vi "E816_Piezo_ctrl_Sereial_mvmnt.vi"() -> ()   [LabVIEW 2016]
doc: "This VI demonstrates how to initialize an E-816 system, how to move an axis and how to query for the position value of this axis.\n\nIn this example the E-816 is connected through COM port 1 with baudrate 57600. The VI runs E816_Configuration_Setup.vi with these specified settings, moves the first axis relative to its current position, waits for the movement to finish and reads the position of the axis and the error status of the controller. The diagram shows how to combine the driver VIs for these tasks. \n\nFor an example of how to command multiple axes through an USB connection see E816_Sample_ Application_1a.vi\n\nWarning: Before running this VI, modify the interface settings on the block diagram to reflect your configuration. The predefined settings provided with the VI probably do not match your system."
panel:
  out "Position":dbl[](array[numeric]) format="%.6f"
  out "First conn. axis":string[](array[string])
  in  "Step values 2":dbl[](array[numeric])=[0.01]
  in  "move":bool
  in  "stop":bool
  in  "error in":errorcluster
  out "Running":bool caption="Configuration_Setup.vi is running"
  out "error out":errorcluster
  out "Identification":string
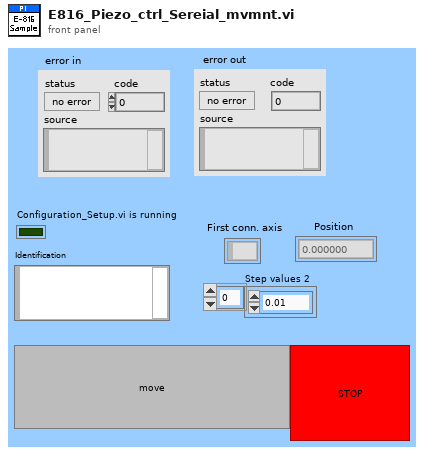
[diagram p1: front panel]
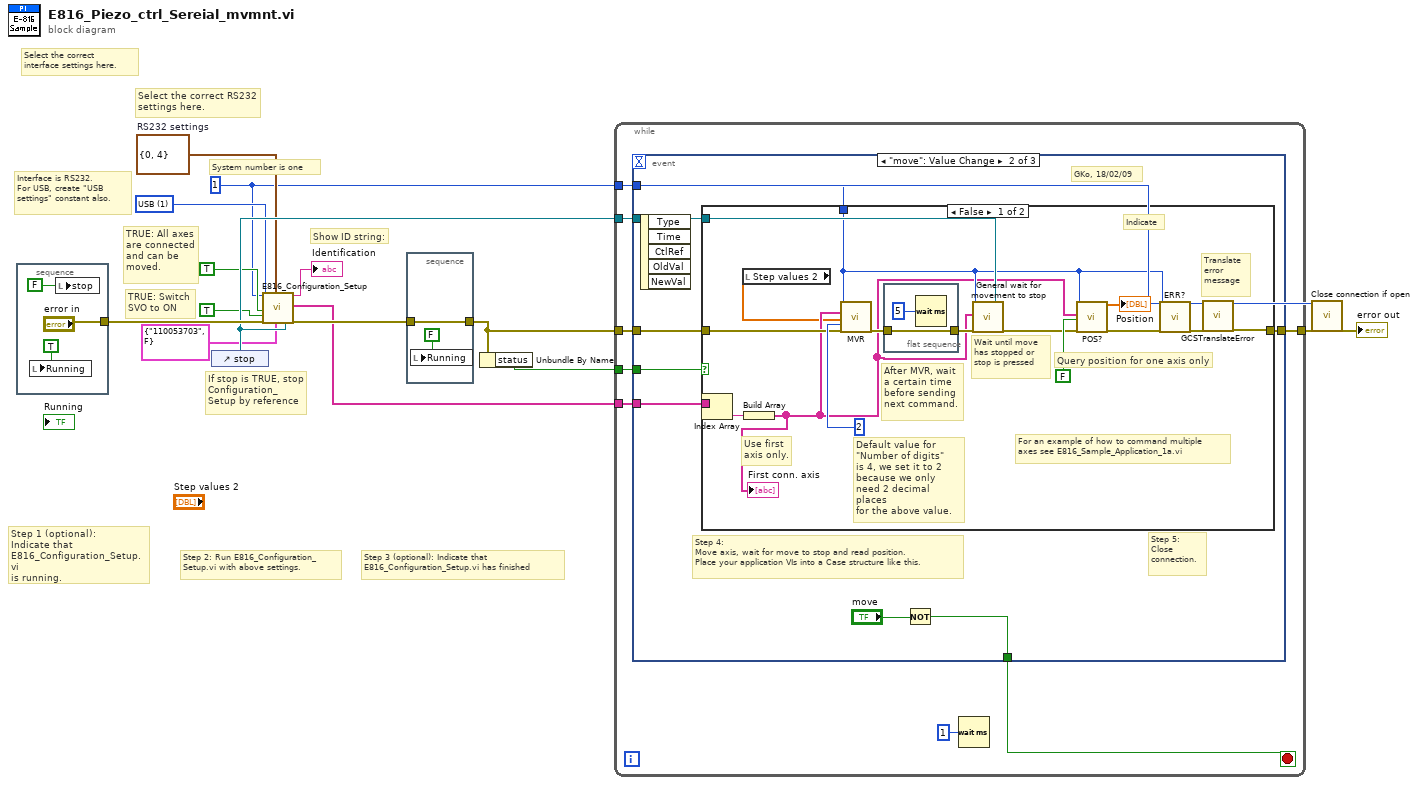
[diagram p0: block diagram]
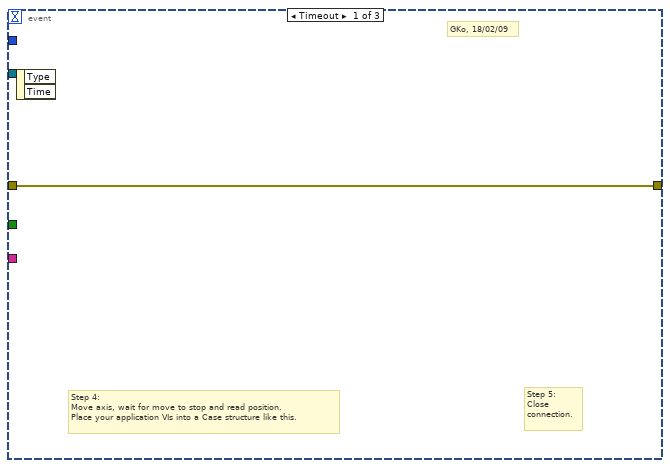
[diagram p2: hidden frame]
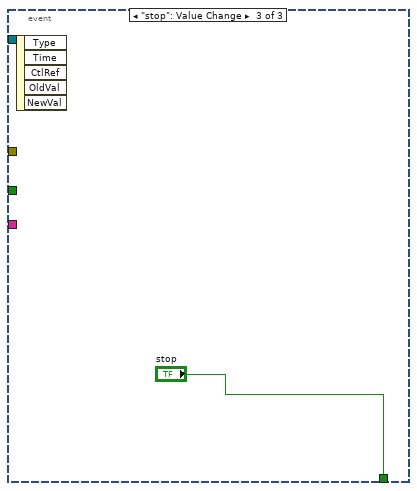
[diagram p4: hidden frame]
diagram:
  w5 = u16 1 items=["RS232", "USB"] ("Interface")
  w8 = cluster{"Portnumber":i32, "Baudrate":u16} {"Portnumber"=0, "Baudrate"=4}  # RS232 settings
  w2 = 1 ("System no.")
  # "Select the correct\ninterface settings here."
  # "Interface is RS232.\nFor USB, create \"USB\nsettings\" constant also."
  # "TRUE: All axes\nare connected\nand can be\nmoved."
  # "TRUE: Switch\nSVO to ON"
  # "If stop is TRUE, stop\nConfiguration_\nSetup by reference"
  # "Select the correct RS232\nsettings here."
  # "Step 3 (optional): Indicate that \nE816_Configuration_Setup.vi has finished"
  # "Step 2: Run E816_Configuration_\nSetup.vi with above settings."
  # "Step 1 (optional): \nIndicate that \nE816_Configuration_Setup.vi\nis running."
  # "Show ID string:"
  # "System number is one"
  n1 = stacked-sequence {
    tunnel: ["error in"] -> w13
    frame #0 {
      n2 = local write "Running"(TRUE ("Running")) -> ()
      n3 = local write "stop"(FALSE ("stop")) -> ()
    }
  }
  n4 = control-ref of="stop"() -> (w10:refnum<vi>)
  n5 = call "E816_Configuration_Setup.vi"("System no."=w2, "Interface"=w5, "All axes?"=TRUE, "Change servo \nstatus to ON?"=TRUE ("Use dialog to define\nconnected stages?"), "error in"=w13, "RS232 settings"=w8, "USB settings"=cluster{"S/N":string, "USB Search?":bool} {"S/N"="110053703", "USB Search?"=FALSE}, "Stop refnum"=w10) -> ("Identification"=→"Identification":string, "Conn. Axes"=w9:string[], "error out"=w14:errorcluster)  [unwired: 3 in, 6 out]
  n6 = stacked-sequence {
    tunnel: w14 -> [w20]
    tunnel: [w20] -> w12
    frame #0 {
      n7 = local write "Running"(FALSE ("Running")) -> ()
    }
  }
  n8 = Unbundle By Name(w12) -> ("status"=w11:bool)
  n9 = while {
    tunnel: w12 -> [w28]
    tunnel: w11 -> [w27]
    tunnel: w10 -> [w26]
    tunnel: w9 -> [w25]
    tunnel: [w24] -> w4
    tunnel: w2 -> [w23]
    stop <- w22 stop-if-true
    n10 = event shown="[1] \"move\": Value Change" {
      selector: _ -> [_ _ _]
      dyn-events: _ -> [_ _ _]
      timeout: _ -> [_ _ _]
      tunnel: w28 -> [w29 w37 _]
      tunnel: w27 -> [_ w36 _]
      tunnel: w26 -> [_ w35 _]
      tunnel: w25 -> [_ w34 _]
      tunnel: [w29 w33 _] -> w24
      tunnel: w23 -> [_ w32 _]
      tunnel: [_ w30 "stop"] -> w22
      event Timeout {
        # "Step 5: \nClose\nconnection."
        # "Step 4: \nMove axis, wait for move to stop and read position.\nPlace your application VIs into a Case structure like this."
        # "GKo, 18/02/09"
        n11 = event-data() -> ()  [unwired: 1 in, 2 out]
      }
      event "move": Value Change {
        # "Step 5: \nClose\nconnection."
        # "Step 4: \nMove axis, wait for move to stop and read position.\nPlace your application VIs into a Case structure like this."
        # "GKo, 18/02/09"
        n12 = event-data() -> ()  [unwired: 1 in, 5 out]
        n13 = case shown="False" w36 {
          tunnel: [w51 w57] -> w33
          tunnel: w34 -> [w43 _]
          tunnel: w32 -> [w47 _]
          tunnel: w37 -> [w52 w57]
          tunnel: w35 -> [w50 _]
          frame False {
            # "For an example of how to command multiple\naxes see E816_Sample_Application_1a.vi"
            # "Use first\naxis only."
            # "After MVR, wait\na certain time\nbefore sending\nnext command."
            # "Translate\nerror \nmessage"
            # "Wait until move\nhas stopped or\nstop is pressed"
            # "Indicate"
            # "Default value for\n\"Number of digits\"\nis 4, we set it to 2\nbecause we only\nneed 2 decimal places\nfor the above value."
            # "Query position for one axis only"
            n14 = Index Array(array=w43, index=0) -> (element=w41:string)
            n15 = local read "Step values 2"() -> (w38:dbl[])
            n16 = Build Array(w41) -> (w40:string[])
            "First conn. axis" <- w40
            n17 = call "MVR.vi"("System no."=w47, "Axes to move"=w40, "Position values"=w38, "No.of digits"=i16 2, "error in"=w52) -> ("error out"=w45:errorcluster)  [unwired: 14 out]
            n18 = flat-sequence {
              tunnel: w45 -> [w56]
              tunnel: [w56] -> w44
              frame #0 {
                n19 = Wait (ms)(milliseconds to wait=u32 5) -> ()  [unwired: 1 out]
              }
            }
            n20 = call "General wait for movement to stop.vi"("System no."=w47, "Axes to wait for"=w40, "error in"=w44, "Stop refnum"=w50) -> ("error out"=w46:errorcluster)  [unwired: 4 in, 11 out]
            n21 = call "POS?.vi"("System no."=w47, "Axes to query"=w40, "All axes?"=FALSE, "error in"=w46) -> ("Position"=→"Position":dbl[], "error out"=w49:errorcluster)  [unwired: 1 in, 13 out]
            n22 = call "ERR?.vi"("System no."=w47, "error in"=w49) -> ("error out"=w48:errorcluster)  [unwired: 17 out]
            n23 = call "GCSTranslateError.vi"("error in"=w48) -> ("error out"=w51:errorcluster)  [unwired: 18 out]
          }
          frame True {
            # "Error during initialization"
          }
        }
        n24 = Not(x="move") -> (.not. x?=w30:bool)
      }
      event "stop": Value Change {
        n25 = event-data() -> ()  [unwired: 1 in, 5 out]
      }
    }
    n26 = Wait (ms)(milliseconds to wait=u32 1) -> ()  [unwired: 1 out]
  }
  n27 = call "Close connection if open.vi"("System no."=w2, "error in"=w4) -> ("error out"=→"error out":errorcluster)  [unwired: 1 in, 16 out]
